vi "nanocal -- nuclear schottky fit V8.vi"() -> ()   [LabVIEW 2021] (continued)
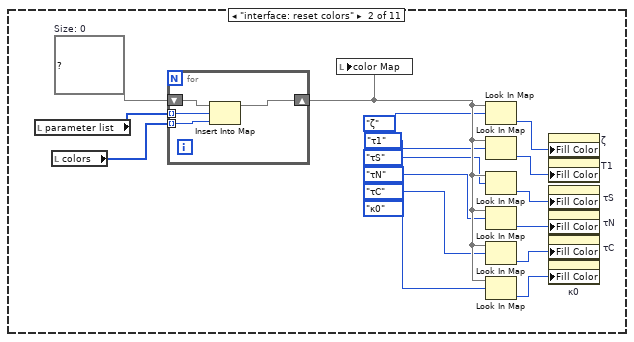
[diagram p3: hidden frame]
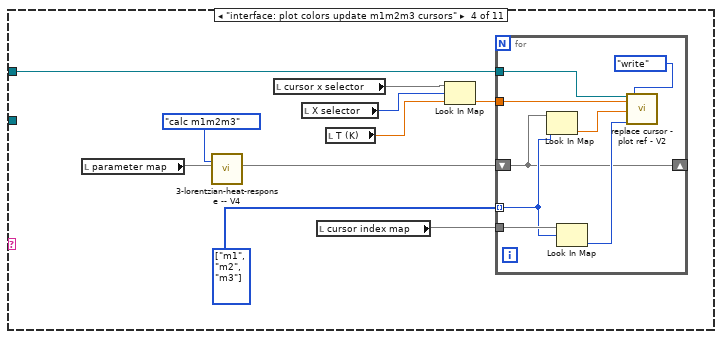
[diagram p4: hidden frame]
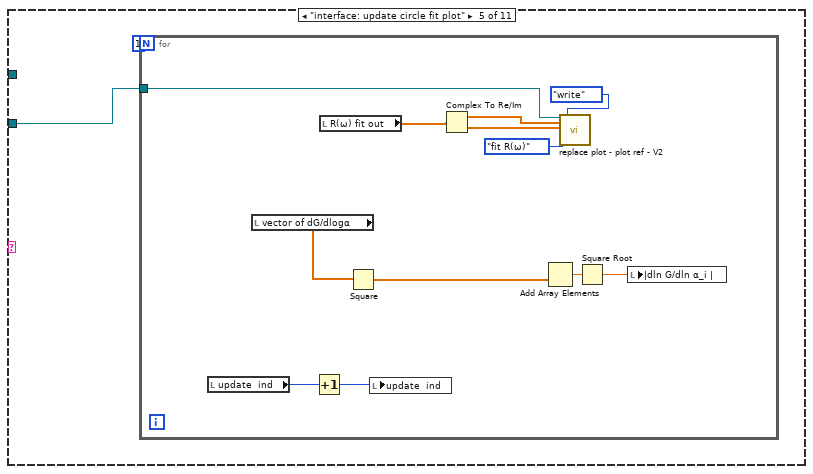
[diagram p5: hidden frame]
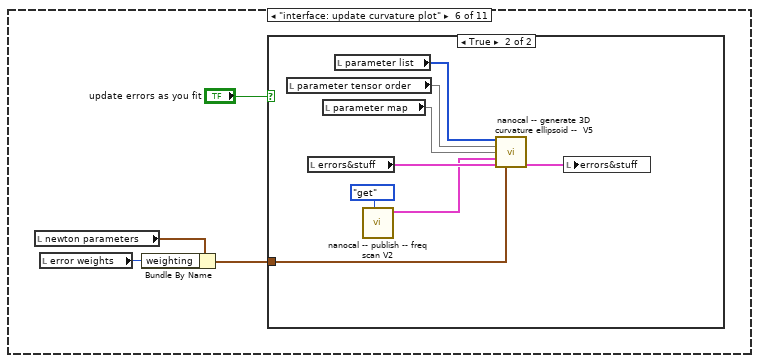
[diagram p6: hidden frame]
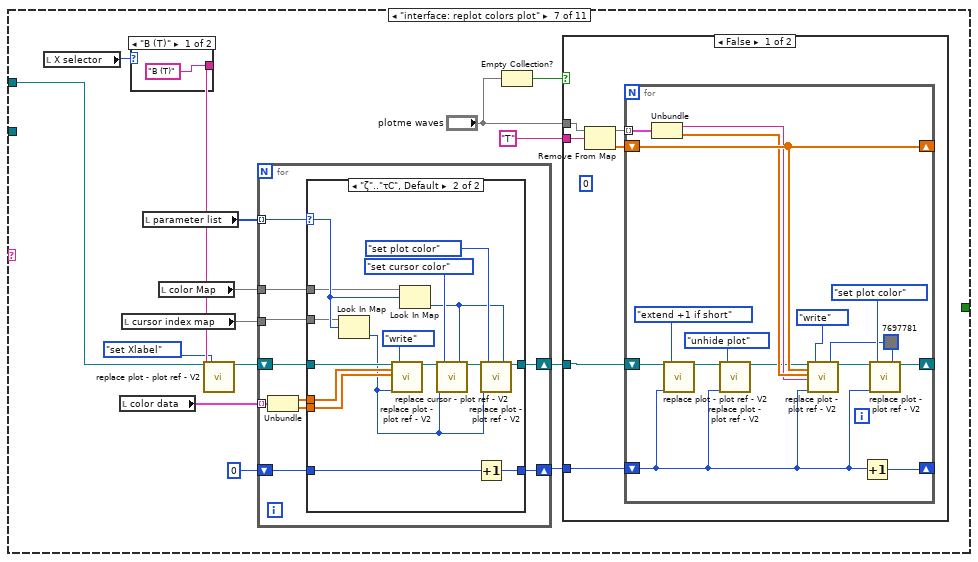
[diagram p8: hidden frame]
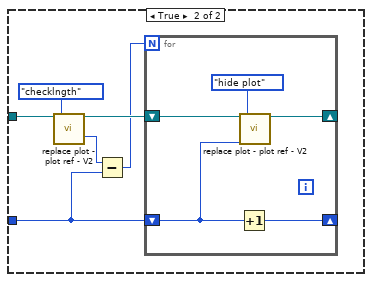
[diagram p9: hidden frame]
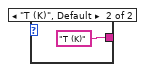
[diagram p10: hidden frame]
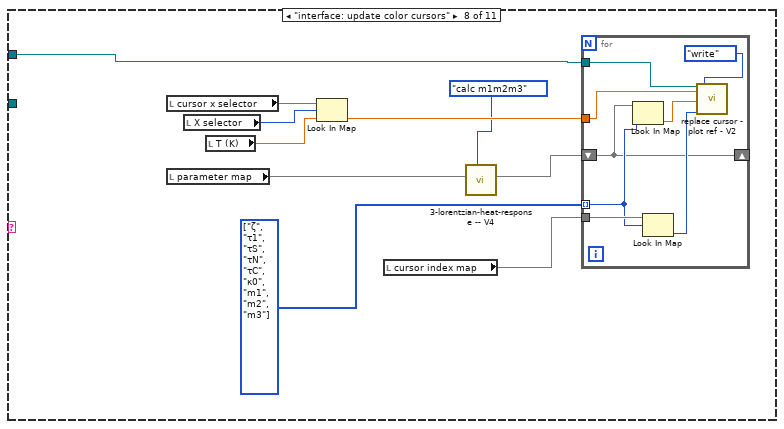
[diagram p12: hidden frame]
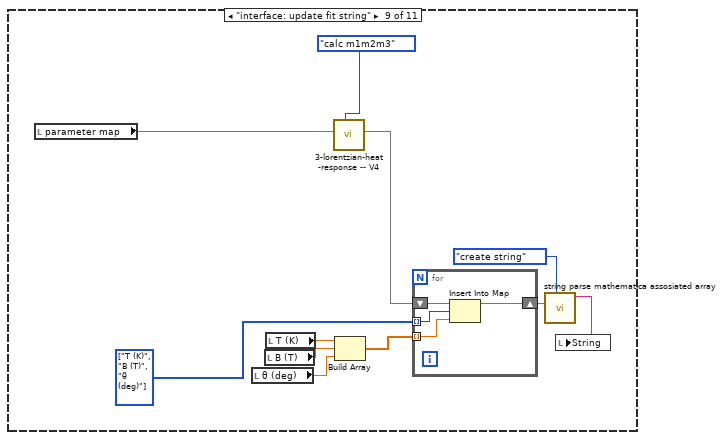
[diagram p13: hidden frame]
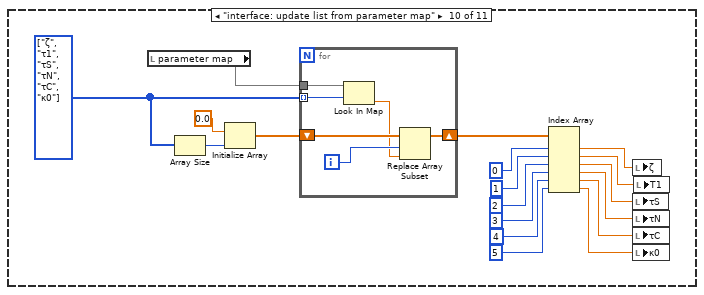
[diagram p14: hidden frame]
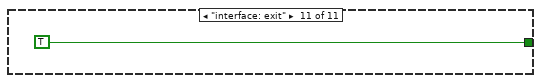
[diagram p15: hidden frame]
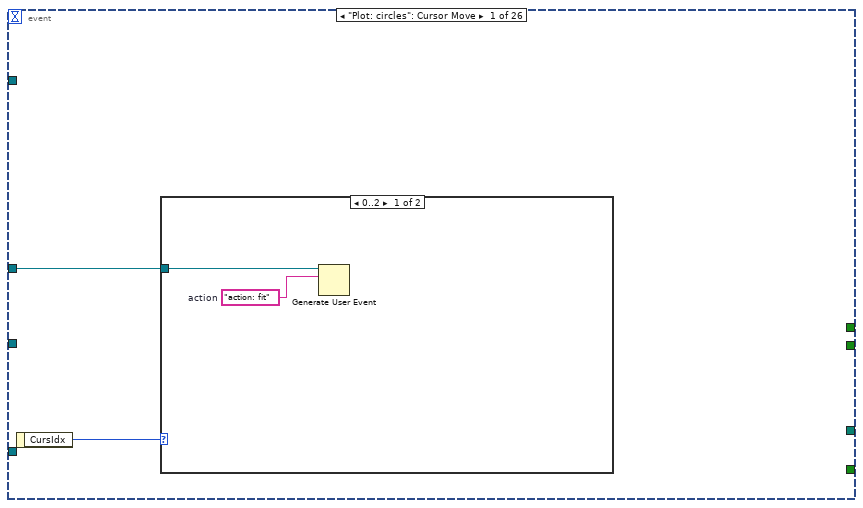
[diagram p16: hidden frame]
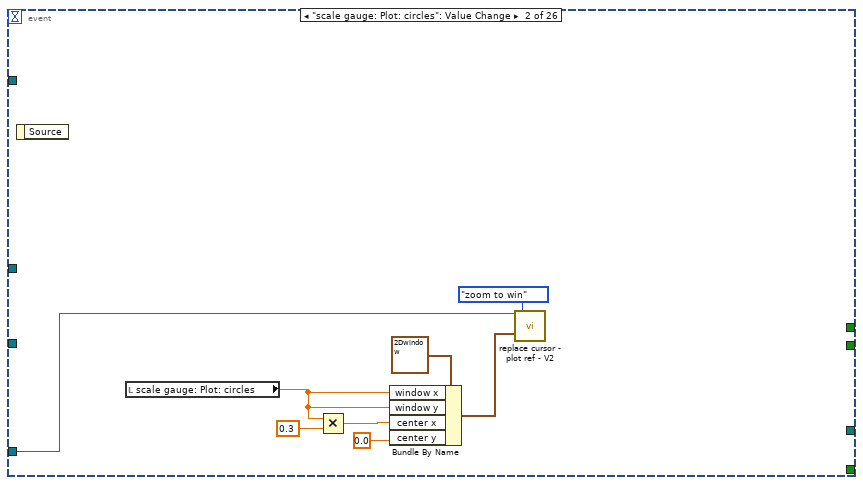
[diagram p18: hidden frame]
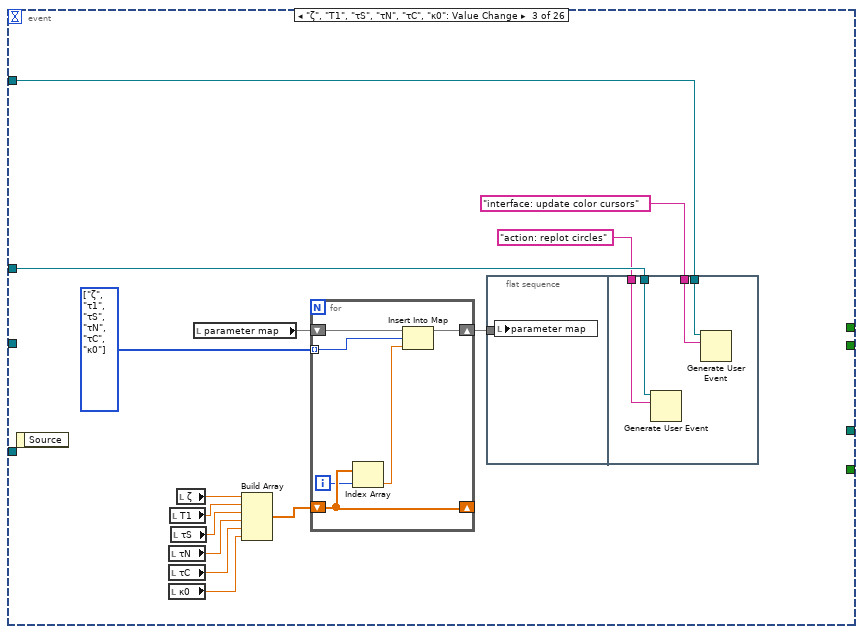
[diagram p19: hidden frame]
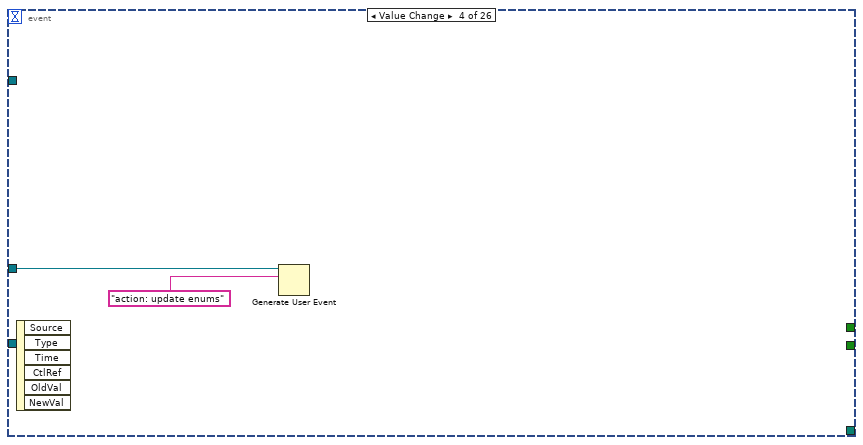
[diagram p20: hidden frame]
        n793 = call "replace cursor - plot ref - V2.vi"("Plot ref in"=w1635, "cursor index"=w1633, "cursor action"=cursor_action."read") -> ("read Y"=w1632:dbl)  [unwired: 13 in, 3 out]
        n794 = local read "parameter map"() -> (w1631:map{T1, dbl})
        n795 = Look In Map(map=w1634, key=w1633) -> (value=w1629:T1)  [unwired: 1 in, 1 out]
        n796 = in-place {
          in-place-border: w1632 -> [w1643]
          in-place-border: LVMapReplaceAction."Modify Entry only if found" ("action") -> [w1642]
          n797 = in-place-map #10(w1631, w1629) -> ()  [unwired: 1 in, 2 out]
          n798 = in-place-map #10(w1643, w1642) -> (w1630:map{T1, dbl})  [unwired: 2 out]
        }
        n799 = flat-sequence {
          tunnel: w1630 -> [w1637]
          tunnel: w1627 -> [w1641]
          tunnel: "action: replot circles" ("event data") -> [w1640]
          tunnel: w1625 -> [w1639]
          tunnel: "interface: update list from parameter map" ("event data") -> [w1638]
          frame #0 {
            n800 = local write "parameter map"(w1637) -> ()
          }
          frame #1 {
            n801 = Generate User Event(user event=w1641, event data cluster=w1640) -> ()  [unwired: 2 in, 2 out]
            n802 = Generate User Event(user event=w1639, event data cluster=w1638) -> ()  [unwired: 2 in, 2 out]
          }
        }
      }
      event "Plot:  colors": Cursor Release {
        n803 = event-data() -> ("CursIdx"=w1654:i32)  [unwired: 1 in]
        n804 = local read "reverse cursor index map"() -> (w1655:map{i32, T1})
        n805 = call "replace cursor - plot ref - V2.vi"("Plot ref in"=w1656, "cursor index"=w1654, "cursor action"=cursor_action."read") -> ("read Y"=w1653:dbl)  [unwired: 13 in, 3 out]
        n806 = local read "parameter map"() -> (w1652:map{T1, dbl})
        n807 = Look In Map(map=w1655, key=w1654) -> (value=w1650:T1)  [unwired: 1 in, 1 out]
        n808 = in-place {
          in-place-border: w1653 -> [w1666]
          in-place-border: LVMapReplaceAction."Modify Entry only if found" ("action") -> [w1665]
          n809 = in-place-map #11(w1652, w1650) -> ()  [unwired: 1 in, 2 out]
          n810 = in-place-map #11(w1666, w1665) -> (w1651:map{T1, dbl})  [unwired: 2 out]
        }
        n811 = flat-sequence {
          tunnel: w1651 -> [w1658]
          tunnel: w1648 -> [w1664]
          tunnel: "action: replot circles" ("event data") -> [w1663]
          tunnel: w1646 -> [w1662]
          tunnel: "interface: update list from parameter map" ("event data") -> [w1661]
          tunnel: "interface: plot colors update m1m2m3 cursors" ("event data") -> [w1659]
          frame #0 {
            n812 = local write "parameter map"(w1658) -> ()
          }
          frame #1 {
            n813 = Generate User Event(user event=w1664, event data cluster=w1663) -> ()  [unwired: 2 in, 2 out]
            n814 = Generate User Event(user event=w1662, event data cluster=w1661) -> (user event out=w1660:refnum<user-event>)  [unwired: 2 in, 1 out]
            n815 = Generate User Event(user event=w1660, event data cluster=w1659) -> ()  [unwired: 2 in, 2 out]
          }
        }
      }
      event "Math→τ! :q": Value Change {
        n816 = event-data() -> ()  [unwired: 1 in, 1 out]
        n817 = Generate User Event(user event=w1668, event data cluster="action: copy from math" ("event data")) -> ()  [unwired: 2 in, 2 out]
      }
      event "load defaults": Value Change {
        n818 = event-data() -> ()  [unwired: 1 in, 1 out]
        n819 = Generate User Event(user event=w1670, event data cluster="action: update default values" ("event data")) -> ()  [unwired: 2 in, 2 out]
      }
      event "τ→Math! :p": Value Change {
        n820 = event-data() -> ()  [unwired: 1 in, 1 out]
        n821 = Generate User Event(user event=w1674, event data cluster="action: copy to math" ("event data")) -> ()  [unwired: 2 in, 2 out]
      }
      event "Math→ string OUT! :s": Value Change {
        n822 = event-data() -> ()  [unwired: 1 in, 1 out]
        n823 = Generate User Event(user event=w1677, event data cluster="action: write mathematica string" ("event data")) -> ()  [unwired: 2 in, 2 out]
      }
      event "generate empty string from filelist !": Value Change {
        n824 = event-data() -> ()  [unwired: 1 in, 1 out]
        n825 = Generate User Event(user event=w1680, event data cluster="action: empty string from filelist" ("event data")) -> ()  [unwired: 2 in, 2 out]
      }
      event "string IN → Math! :~": Value Change {
        n826 = event-data() -> ()  [unwired: 1 in, 1 out]
        n827 = Generate User Event(user event=w1683, event data cluster="action: read mathematica string" ("event data")) -> ()  [unwired: 2 in, 2 out]
      }
      event "filenames": Value Change {
        n828 = event-data() -> ()  [unwired: 1 in, 1 out]
        n829 = local read "filesnames lookup"() -> (w1690:map{i32, string})
        n830 = local read "all full filenames"() -> (w1688:map{string, path})
        n831 = local read "filenames"() -> (w1689:u16)
        n832 = Look In Map(map=w1690, key=w1689) -> (value=w1687:string)  [unwired: 1 in, 1 out]
        n833 = Look In Map(map=w1688, key=w1687) -> (value=w1685:path)  [unwired: 1 in, 1 out]
        n834 = for {
          N: 1 -> [_]
          tunnel: w1691 -> [w1693]
          tunnel: w1685 -> [w1692]
          n835 = local write "Read from file"(w1692) -> ()
          n836 = Generate User Event(user event=w1693, event data cluster="action: read from file" ("event data")) -> ()  [unwired: 2 in, 2 out]
        }
      }
      event "selection :|\\": Value Change {
        n837 = event-data() -> ()  [unwired: 1 in, 1 out]
        n838 = Generate User Event(user event=w1695, event data cluster="action: constrained filenames select" ("event data")) -> ()  [unwired: 2 in, 2 out]
      }
      event "plot landscape!", "range one", "range two": Value Change {
        n839 = event-data() -> ()  [unwired: 1 in, 6 out]
        n840 = Generate User Event(user event=w1697, event data cluster="action: plot landscape" ("event data")) -> ()  [unwired: 2 in, 2 out]
      }
      event "colors": Value Change {
        n841 = event-data() -> ()  [unwired: 1 in, 6 out]
        n842 = Generate User Event(user event=w1700, event data cluster="action: reset colors" ("event data")) -> ()  [unwired: 2 in, 2 out]
      }
    }
  }
  "cursor x selector" <- w43
